vi "量程参数写入.vi"(7 "量程切换阈值":cluster{"阈值":dbl, "标液浓度":dbl}, 8 "error in (no error)":errorcluster, 9 "量程下拉列表":enum16{"低量程", "高量程"}(ring), 10 "测量模式":enum16{"跨度核查", "水样测量", "零点核查", "标样核查", "加标回收"}(ring), 11 "参数下拉列表":u16(ring) items=["总磷"=1, "总氮"=2]) -> (0 "error out":errorcluster)   [LabVIEW 2016, in "斯坦道总氮V2.lvlib"]
uses:
  <vilib>/Utility/error.llb/Error Cluster From Error Code.vi
  <vilib>/ErrorRing/Error Ring.xnode
  <vilib>/Plasmionique/MB Master/MB Master.lvlib
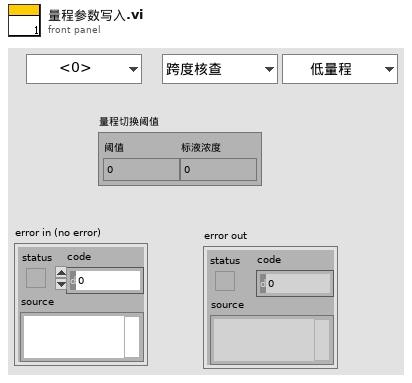
[diagram p1: front panel]
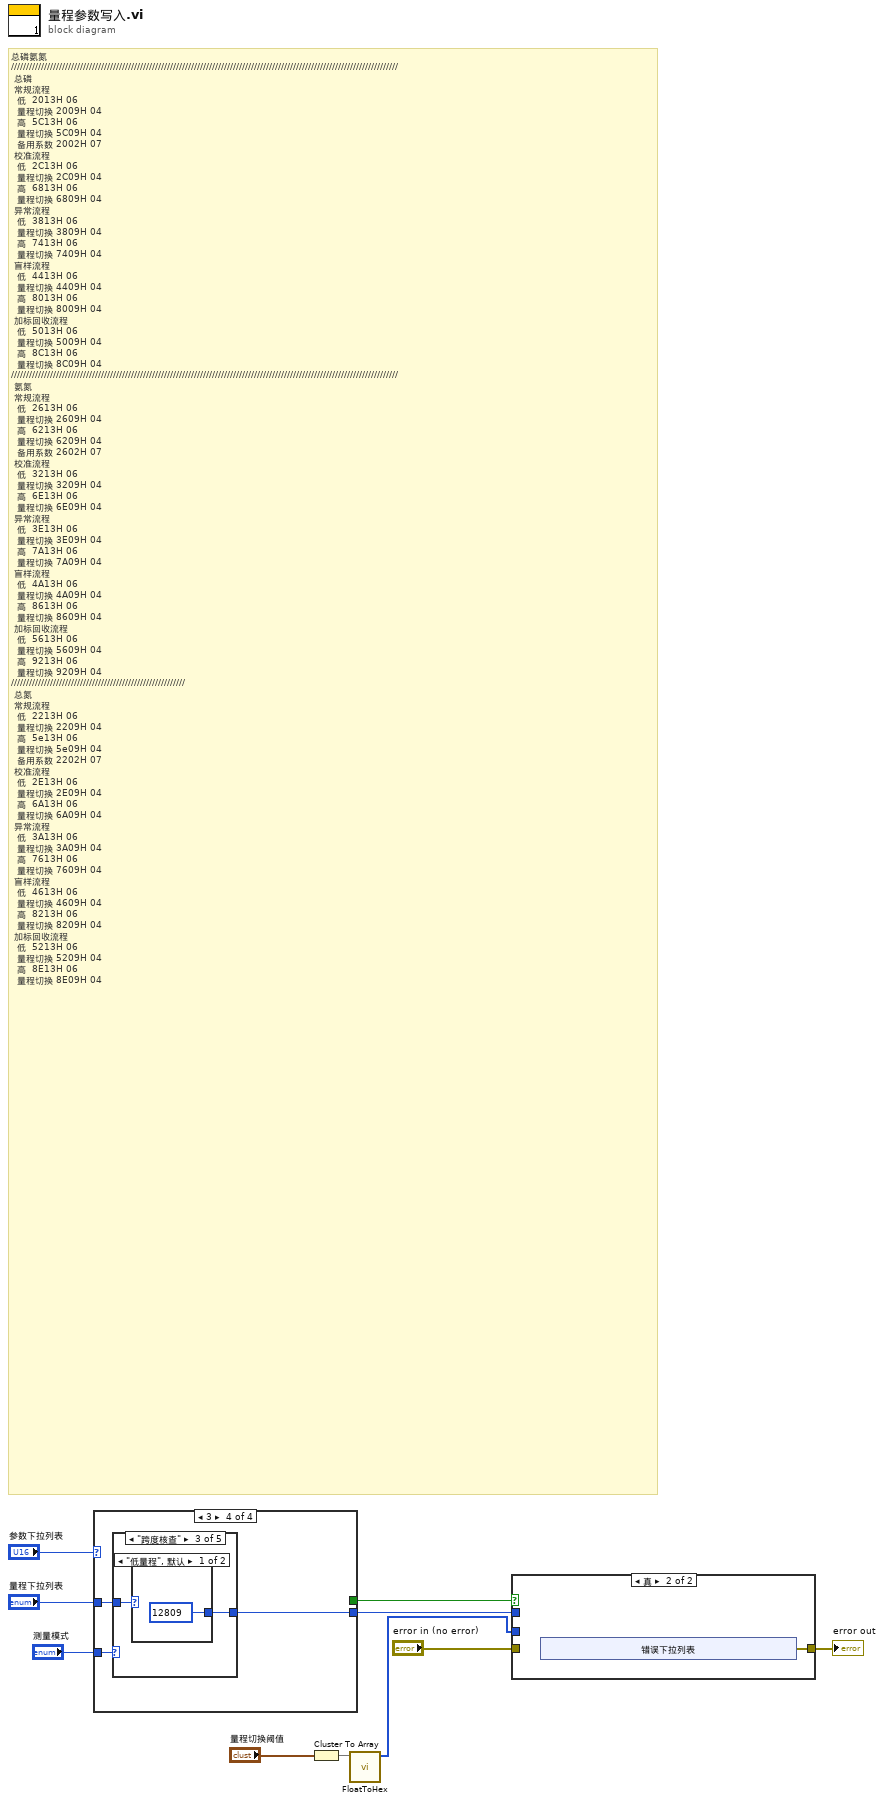
[diagram p0: block diagram]
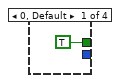
[diagram p2: hidden frame]
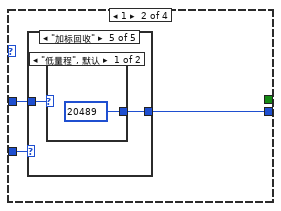
[diagram p3: hidden frame]
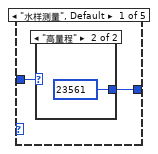
[diagram p4: hidden frame]
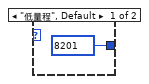
[diagram p5: hidden frame]
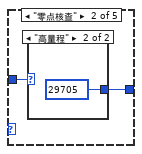
[diagram p6: hidden frame]
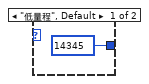
[diagram p7: hidden frame]
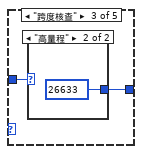
[diagram p8: hidden frame]
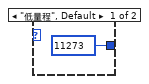
[diagram p9: hidden frame]
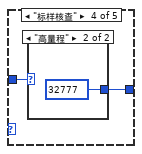
[diagram p10: hidden frame]
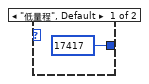
[diagram p11: hidden frame]
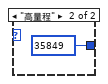
[diagram p12: hidden frame]
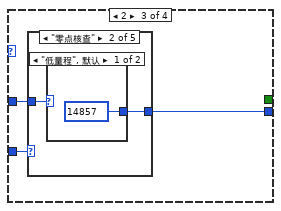
[diagram p13: hidden frame]
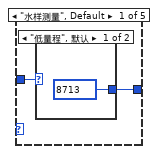
[diagram p14: hidden frame]
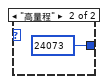
[diagram p15: hidden frame]
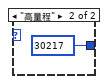
[diagram p16: hidden frame]
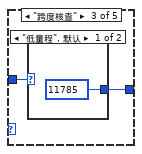
[diagram p17: hidden frame]
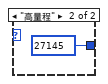
[diagram p18: hidden frame]
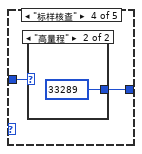
[diagram p19: hidden frame]
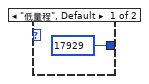
[diagram p20: hidden frame]
diagram:
  # "总磷氨氮\n/////////////////////////////////////////////////////////////////////////////////////////////////////////////////////////////////\n\t总磷\n\t常规流程\n\t\t低\t\t2013H\t06\n\t\t量程切换\t2009H\t04\n\t\t高\t\t5C13H\t06\n\t\t量程切换\t5C09H\t04\n\t\t备用系数\t2002H\t07\n\t校准流程\n\t\t低\t\t2C13H\t06\n\t\t量程切换\t2C09H\t04\n\t\t高\t\t6813H\t06\n\t\t量程切换\t6809H\t04\n\t异常流程\n\t\t低\t\t3813H\t06\n\t\t量程切换\t3809H\t04\n\t\t高\t\t7413H\t06\n\t\t量程切换\t7409H\t04\t\n\t盲样流程\n\t\t低\t\t4413H\t06\n\t\t量程切换\t4409H\t04\n\t\t高\t\t8013H\t06\n\t\t量程切换\t8009H\t04\t\n\t加标回收流程\n\t\t低\t\t5013H\t06\n\t\t量程切换\t5009H\t04\n\t\t高\t\t8C13H\t06\n\t\t量程切换\t8C09H\t04\t\n/////////////////////////////////////////////////////////////////////////////////////////////////////////////////////////////////\n\t氨氮\n\t常规流程\n\t\t低\t\t2613H\t06\n\t\t量程切换\t2609H\t04\n\t\t高\t\t6213H\t06\n\t\t量程切换\t6209H\t04\n\t\t备用系数\t2602H\t07\n\t校准流程\n\t\t低\t\t3213H\t06\n\t\t量程切换\t3209H\t04\n\t\t高\t\t6E13H\t06\n\t\t量程切换\t6E09H\t04\n\t异常流程\n\t\t低\t\t3E13H\t06\n\t\t量程切换\t3E09H\t04\n\t\t高\t\t7A13H\t06\n\t\t量程切换\t7A09H\t04\t\n\t盲样流程\n\t\t低\t\t4A13H\t06\n\t\t量程切换\t4A09H\t04\n\t\t高\t\t8613H\t06\n\t\t量程切换\t8609H\t04\t\n\t加标回收流程\n\t\t低\t\t5613H\t06\n\t\t量程切换\t5609H\t04\n\t\t高\t\t9213H\t06\n\t\t量程切换\t9209H\t04\t\n//////////////////////////////////////////////////////////\n\t总氮\n\t常规流程\n\t\t低\t\t2213H\t06\n\t\t量程切换\t2209H\t04\n\t\t高\t\t5e13H\t06\n\t\t量程切换\t5e09H\t04\n\t\t备用系数\t2202H\t07\n\t校准流程\n\t\t低\t\t2E13H\t06\n\t\t量程切换\t2E09H\t04\n\t\t高\t\t6A13H\t06\n\t\t量程切换\t6A09H\t04\n\t异常流程\n\t\t低\t\t3A13H\t06\n\t\t量程切换\t3A09H\t04\n\t\t高\t\t7613H\t06\n\t\t量程切换\t7609H\t04\t\n\t盲样流程\n\t\t低\t\t4613H\t06\n\t\t量程切换\t4609H\t04\n\t\t高\t\t8213H\t06\n\t\t量程切换\t8209H\t04\t\n\t加标回收流程\n\t\t低\t\t5213H\t06\n\t\t量程切换\t5209H\t04\n\t\t高\t\t8E13H\t06\n\t\t量程切换\t8E09H\t04"
  n1 = case shown="3" "参数下拉列表" {
    tunnel: "测量模式" -> [_ w14 w37 w60]
    tunnel: "量程下拉列表" -> [_ w13 w36 w59]
    tunnel: [_ w12 w35 w58] -> w3
    tunnel: [TRUE _ _ _] -> w2
    frame 0, Default {
    }
    frame 1 {
      n2 = case shown="\"加标回收\"" w14 {
        tunnel: w13 -> [w16 w20 w24 w28 w32]
        tunnel: [w15 w19 w23 w27 w31] -> w12
        frame "水样测量", Default {
          n3 = case shown="\"高量程\"" w16 {
            tunnel: [u16 8201 ("starting address") u16 23561 ("starting address")] -> w15
            frame "低量程", Default {
            }
            frame "高量程" {
            }
          }
        }
        frame "零点核查" {
          n4 = case shown="\"高量程\"" w20 {
            tunnel: [u16 14345 ("starting address") u16 29705 ("starting address")] -> w19
            frame "低量程", Default {
            }
            frame "高量程" {
            }
          }
        }
        frame "跨度核查" {
          n5 = case shown="\"高量程\"" w24 {
            tunnel: [u16 11273 ("starting address") u16 26633 ("starting address")] -> w23
            frame "低量程", Default {
            }
            frame "高量程" {
            }
          }
        }
        frame "标样核查" {
          n6 = case shown="\"高量程\"" w28 {
            tunnel: [u16 17417 ("starting address") u16 32777 ("starting address")] -> w27
            frame "低量程", Default {
            }
            frame "高量程" {
            }
          }
        }
        frame "加标回收" {
          n7 = case shown="\"低量程\", 默认" w32 {
            tunnel: [u16 20489 ("starting address") u16 35849 ("starting address")] -> w31
            frame "低量程", Default {
            }
            frame "高量程" {
            }
          }
        }
      }
    }
    frame 2 {
      n8 = case shown="\"零点核查\"" w37 {
        tunnel: w36 -> [w39 w43 w47 w51 w55]
        tunnel: [w38 w42 w46 w50 w54] -> w35
        frame "水样测量", Default {
          n9 = case shown="\"低量程\", 默认" w39 {
            tunnel: [u16 8713 ("starting address") u16 24073 ("starting address")] -> w38
            frame "低量程", Default {
            }
            frame "高量程" {
            }
          }
        }
        frame "零点核查" {
          n10 = case shown="\"低量程\", 默认" w43 {
            tunnel: [u16 14857 ("starting address") u16 30217 ("starting address")] -> w42
            frame "低量程", Default {
            }
            frame "高量程" {
            }
          }
        }
        frame "跨度核查" {
          n11 = case shown="\"低量程\", 默认" w47 {
            tunnel: [u16 11785 ("starting address") u16 27145 ("starting address")] -> w46
            frame "低量程", Default {
            }
            frame "高量程" {
            }
          }
        }
        frame "标样核查" {
          n12 = case shown="\"高量程\"" w51 {
            tunnel: [u16 17929 ("starting address") u16 33289 ("starting address")] -> w50
            frame "低量程", Default {
            }
            frame "高量程" {
            }
          }
        }
        frame "加标回收" {
          n13 = case shown="\"低量程\", 默认" w55 {
            tunnel: [u16 21001 ("starting address") u16 36361 ("starting address")] -> w54
            frame "低量程", Default {
            }
            frame "高量程" {
            }
          }
        }
      }
    }
    frame 3 {
      n14 = case shown="\"跨度核查\"" w60 {
        tunnel: w59 -> [w62 w66 w70 w74 w78]
        tunnel: [w61 w65 w69 w73 w77] -> w58
        frame "水样测量", Default {
          n15 = case shown="\"高量程\"" w62 {
            tunnel: [u16 9737 ("starting address") u16 25097 ("starting address")] -> w61
            frame "低量程", Default {
            }
            frame "高量程" {
            }
          }
        }
        frame "零点核查" {
          n16 = case shown="\"低量程\", 默认" w66 {
            tunnel: [u16 15881 ("starting address") u16 31241 ("starting address")] -> w65
            frame "低量程", Default {
            }
            frame "高量程" {
            }
          }
        }
        frame "跨度核查" {
          n17 = case shown="\"低量程\", 默认" w70 {
            tunnel: [u16 12809 ("starting address") u16 28169 ("starting address")] -> w69
            frame "低量程", Default {
            }
            frame "高量程" {
            }
          }
        }
        frame "标样核查" {
          n18 = case shown="\"高量程\"" w74 {
            tunnel: [u16 18963 ("starting address") u16 34323 ("starting address")] -> w73
            frame "低量程", Default {
            }
            frame "高量程" {
            }
          }
        }
        frame "加标回收" {
          n19 = case shown="\"低量程\", 默认" w78 {
            tunnel: [u16 22025 ("starting address") u16 37385 ("starting address")] -> w77
            frame "低量程", Default {
            }
            frame "高量程" {
            }
          }
        }
      }
    }
  }
  n20 = Cluster To Array(cluster="量程切换阈值") -> (array=w10:dbl[])
  n21 = call "FloatToHex.vi"("浮点数"=w10) -> ("DCBA整形输出"=w9:u16[])  [unwired: 10 in]
  n22 = case shown="真" w2 {
    tunnel: w3 -> [w85 _]
    tunnel: w9 -> [w84 _]
    tunnel: "error in (no error)" -> [w82 _]
    tunnel: [w81 w86] -> w7
    frame False {
      n23 = global read "VAR总磷总氮全局变量.vi" "MB session in"() -> (w83:refnum<class "MB_Master.lvclass">)
      n24 = call <vilib>:"Write Multiple Registers.vi"("error in (no error)"=w82, "values"=w84, "starting address"=w85, "MB session in"=w83) -> ("error out"=w81:errorcluster)  [unwired: 6 in, 1 out]
    }
    frame True {
      n25 = xnode "错误下拉列表"() -> ("错误输出"=w86:errorcluster)
    }
  }
  "error out" <- w7
